vi "Close Sessions.vi"(8 "error in":errorcluster, 11 "measurement context in":refnum<class "MeasurementContext.lvclass">) -> (0 "error out":errorcluster, 3 "measurement context out":refnum<class "MeasurementContext.lvclass">)   [LabVIEW 2020, in "MeasurementLink Measurement Server.lvlib" / "MeasurementContext.lvclass"]
uses:
  MeasurementContext.lvclass
  MeasurementContext.lvclass/MeasurementContext.ctl
  MeasurementLink Session Management/Session Reservation/Session Reservation.lvclass
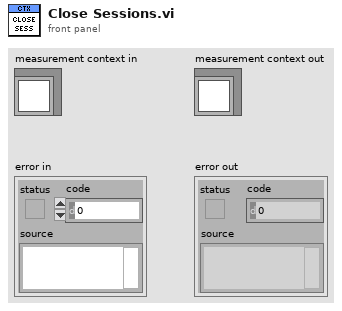
[diagram p1: front panel]
types:
  T1 = typedef "MeasurementLink Measurement Server.lvlib/MeasurementContext.lvclass/Data.ctl" = cluster{"PinMapContext":T2, "gRPCServerId":T3, "IMeasurementService":refnum<class "IMeasurementService.lvclass">, "MeasurementPluginService":refnum<class "MeasurementPluginService.lvclass">, "Session Reservations":refnum<class "Session Reservation.lvclass">[]}
  T2 = typedef "MeasurementLink Measurement Server.lvlib/PinMapContext.ctl" = cluster{"pin_map_id":string, "sites":i32[]}
  T3 = typedef "grpc-lvsupport-release.lvlib/grpcId.ctl" = u64
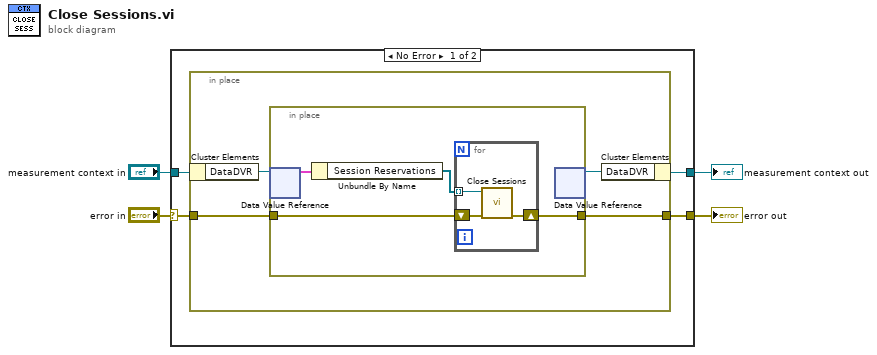
[diagram p0: block diagram]
diagram:
  n1 = case shown="No Error" "error in" {
    selector: "error in" -> [w6 w21]
    tunnel: [w5 w21] -> w3
    tunnel: [w7 w20] -> w1
    tunnel: "measurement context in" -> [w8 w20]
    frame No Error {
      n2 = in-place {
        in-place-border: w6 -> [w10]
        in-place-border: [w9] -> w5
        n3 = in-place-cluster #1(w8) -> ("DataDVR"=w12:refnum<data-value>)
        n4 = in-place {
          in-place-border: w10 -> [w14]
          in-place-border: [w13] -> w9
          n5 = in-place-dvr #2(w12) -> (w16:T1)  [unwired: 1 out]
          n6 = Unbundle By Name(w16) -> ("Session Reservations"=w15:refnum<class "Session Reservation.lvclass">[])
          n7 = for {
            tunnel: w15 -> [w19] mode=indexing
            shift-right: [w17] -> w13
            shift-left: w14 -> [w18]
            n8 = call "Close Sessions.vi"("error in"=w18, "session reservation in"=w19) -> ("error out"=w17:errorcluster)  [unwired: 8 in, 1 out]
          }
          n9 = in-place-dvr #2() -> (w11:refnum<data-value>)  [unwired: 1 in, 1 out]
        }
        n10 = in-place-cluster #1("DataDVR"=w11) -> (w7:refnum<class "MeasurementContext.lvclass">)
      }
    }
    frame Error {
    }
  }
  "error out" <- w3
  "measurement context out" <- w1
